vi "BRig_dataLC_Cue2_PreR_Block_l1.vi"() -> (2 "output_Cue2_PreR_Block":i32)   [LabVIEW 2014]
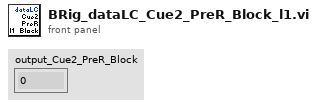
[diagram p1: front panel]
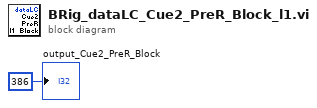
[diagram p0: block diagram]
diagram:
  "output_Cue2_PreR_Block" <- 386 ("output_iBlock")
